vi "Diff Terminals and Acyclic Frames.vi"(5 "port old":T2, 7 "port new":T2, 10 "change type":T1, 11 "refresh items in":T10[](array[typedef])) -> (3 "refresh items out":T10[](array[typedef]))   [LabVIEW 2020, in "AIM MIL-STD-1553 System Explorer.lvlib" / "Implementation.lvlib" / "Refresh.lvlib"]
uses:
  Refresh.lvlib
  MCL Row.ctl
  Change Type.ctl
  Symbols.ctl
  Shared/BIU Configuration.ctl
  Shared/Address.ctl
  Shared/Major Frame Definition.ctl
  Shared/Minor Frame Definition.ctl
  Shared/Message Definition.ctl
  Shared/Message Type.ctl
  Shared/Terminal Endpoint.ctl
  Shared/Parameter Definition.ctl
  Name to Symbol.vi
  Scripting/Constants.vi
  Scripting/AIM MIL-STD-1553 Scripting.lvlib
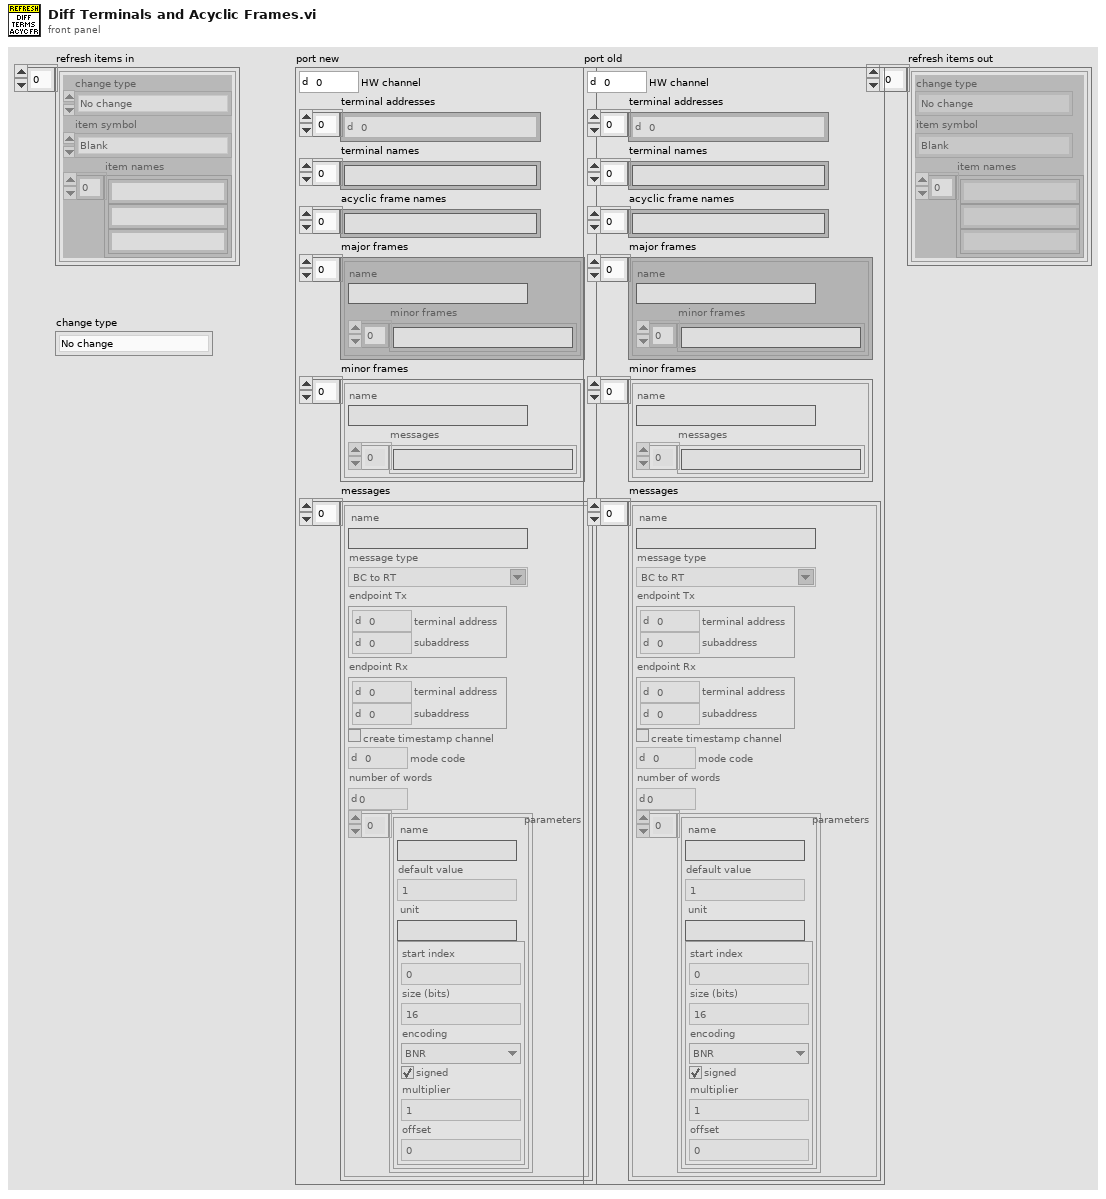
[diagram p1: front panel]
types:
  T1 = typedef "AIM MIL-STD-1553 System Explorer.lvlib/Implementation.lvlib/Refresh.lvlib/Change Type.ctl" = enum16{"No change", "Modify", "Add", "Remove"}
  T2 = typedef "BIU Configuration.ctl" = cluster{"HW channel":u16, "terminal addresses":T3[], "terminal names":string[], "acyclic frame names":string[], "major frames":T4[], "minor frames":T5[], "messages":T6[]}
  T3 = typedef "Address.ctl" = u16
  T4 = typedef "Major Frame Definition.ctl" = cluster{"name":string, "minor frames":string[]}
  T5 = typedef "Minor Frame Definition.ctl" = cluster{"name":string, "messages":string[]}
  T6 = typedef "Message Definition.ctl" = cluster{"name":string, "message type":T7, "endpoint Tx":T8, "endpoint Rx":T8, "create timestamp channel":bool, "mode code":u16, "number of words":u16, "parameters":cluster{"name":string, "default value":dbl, "unit":string, "parameter definition":T9}[]}
  T7 = typedef "Message Type.ctl" = string
  T8 = typedef "Terminal Endpoint.ctl" = cluster{"terminal address":T3, "subaddress":T3}
  T9 = typedef "Parameter Definition.ctl" = cluster{"start index":i32, "size (bits)":i32, "encoding":enum16{"BNR", "BCD", "Discrete"}, "signed":bool, "multiplier":dbl, "offset":dbl}
  T10 = typedef "AIM MIL-STD-1553 System Explorer.lvlib/Implementation.lvlib/Refresh.lvlib/MCL Row.ctl" = cluster{"change type":T1, "item symbol":T11, "item names":string[]}
  T11 = typedef "AIM MIL-STD-1553 System Explorer.lvlib/Implementation.lvlib/Refresh.lvlib/Symbols.ctl" = enum16{"Blank", "MIL-STD-1553", "Port", "Remote Terminal", "Subaddress", "Bus Controller", "Acyclic Frame", "Mode Code", "Message", "Parameter", "Item"}
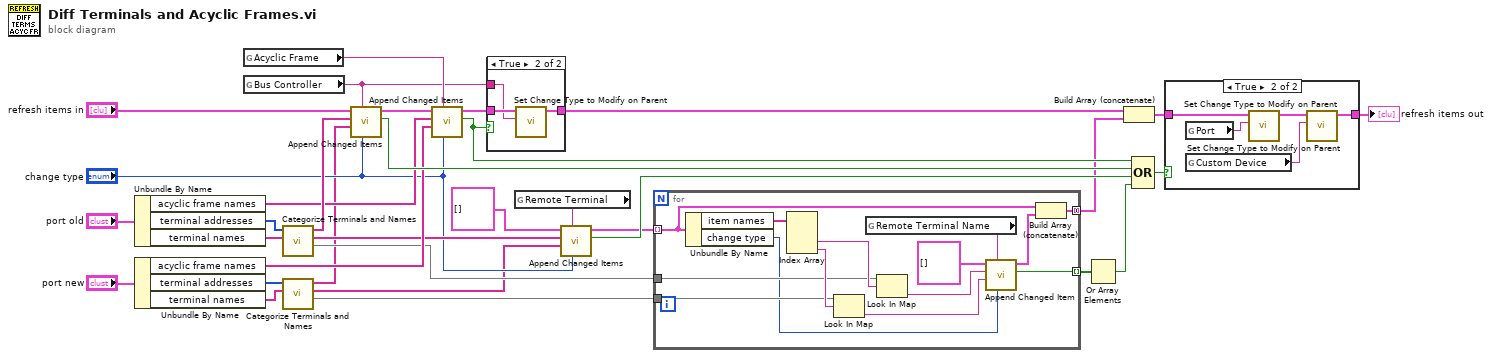
[diagram p0: block diagram]
diagram:
  n1 = Unbundle By Name("port old") -> ("acyclic frame names"=w20:string[], "terminal addresses"=w21:T3[], "terminal names"=w17:string[])
  n2 = Unbundle By Name("port new") -> ("acyclic frame names"=w18:string[], "terminal addresses"=w7:T3[], "terminal names"=w6:string[])
  n3 = global read "Constants.vi" "Acyclic Frame"() -> (w33:string)
  n4 = global read "Constants.vi" "Bus Controller"() -> (w24:string)
  n5 = call "Categorize Terminals and Names.vi"("terminal names"=w17, "terminal addresses"=w21) -> ("map from terminal address (string) to terminal name"=w10:map{string, string}, "remote terminals"=w16:string[], "bus controller"=w30:string[])  [unwired: 7 in]
  n6 = call "Categorize Terminals and Names.vi"("terminal names"=w6, "terminal addresses"=w7) -> ("map from terminal address (string) to terminal name"=w3:map{string, string}, "remote terminals"=w4:string[], "bus controller"=w5:string[])  [unwired: 7 in]
  n7 = call "Append Changed Items.vi"("change type"="change type", "item name"=w24, "items new"=w5, "items old"=w30, "refresh items in"="refresh items in") -> ("modify parent"=w26:bool, "refresh items out"=w31:T10[])  [unwired: 5 in]
  n8 = call "Append Changed Items.vi"("change type"="change type", "item name"=w33, "items new"=w18, "items old"=w20, "refresh items in"=w31) -> ("modify parent"=w27:bool, "refresh items out"=w28:T10[])  [unwired: 5 in]
  n9 = case shown="True" w27 {
    tunnel: w28 -> [w34 w37]
    tunnel: [w34 w36] -> w15
    tunnel: w24 -> [_ w35]
    frame False {
    }
    frame True {
      n10 = call "Set Change Type to Modify on Parent.vi"("parent name"=w35, "refresh items in"=w37) -> ("refresh items out"=w36:T10[])  [unwired: 9 in]
    }
  }
  n11 = global read "Constants.vi" "Remote Terminal"() -> (w32:string)
  n12 = call "Append Changed Items.vi"("change type"="change type", "item name"=w32, "items new"=w4, "items old"=w16, "refresh items in"=T10[] []) -> ("modify parent"=w13:bool, "refresh items out"=w11:T10[])  [unwired: 5 in]
  n13 = for {
    tunnel: w11 -> [w44] mode=indexing
    tunnel: w10 -> [w48]
    tunnel: w3 -> [w47]
    tunnel: [w42] -> w9 mode=indexing
    tunnel: [w41] -> w1 mode=concatenating
    n14 = Unbundle By Name(w44) -> ("item names"=w51:string[], "change type"=w45:T1)
    n15 = Index Array(array=w51) -> (element #2=w50:string, element #3=w49:string)  [unwired: 3 in, 1 out]
    n16 = Look In Map(map=w47, key=w49) -> (value=w39:string)  [unwired: 1 in, 1 out]
    n17 = global read "Constants.vi" "Remote Terminal Name"() -> (w38:string)
    n18 = Look In Map(map=w48, key=w50) -> (value=w46:string)  [unwired: 1 in, 1 out]
    n19 = call "Append Changed Item.vi"("change type"=w45, "item name"=w38, "new value"=w39, "old value"=w46, "refresh items in"=T10[] []) -> ("modify parent"=w42:bool, "refresh items out"=w43:T10[])  [unwired: 5 in]
    n20 = Build Array (concatenate)(w44, w43) -> (w41:T10[])
  }
  n21 = Or Array Elements(Boolean array=w9) -> (logical OR=w2:bool)
  n22 = Build Array (concatenate)(w15, w1) -> (w14:T10[])
  n23 = Compound Arithmetic op=OR(w27, w26, w13, w2) -> (w25:bool)
  n24 = case shown="True" w25 {
    tunnel: w14 -> [w52 w57]
    tunnel: [w52 w54] -> w23
    frame False {
    }
    frame True {
      n25 = global read "Constants.vi" "Port"() -> (w56:string)
      n26 = global read "Constants.vi" "Custom Device"() -> (w53:string)
      n27 = call "Set Change Type to Modify on Parent.vi"("parent name"=w56, "refresh items in"=w57) -> ("refresh items out"=w55:T10[])  [unwired: 9 in]
      n28 = call "Set Change Type to Modify on Parent.vi"("parent name"=w53, "refresh items in"=w55) -> ("refresh items out"=w54:T10[])  [unwired: 9 in]
    }
  }
  "refresh items out" <- w23
